vi "multi_line_to_single_line.vi"(0 "input string":string, 11 "error in (no error)":errorcluster) -> (4 "result string":string, 15 "error out":errorcluster)   [LabVIEW 2023]
doc: "Used to convert a multine string to single line string."
uses:
  <vilib>/Utility/error.llb/Trim Whitespace One-Sided.vi
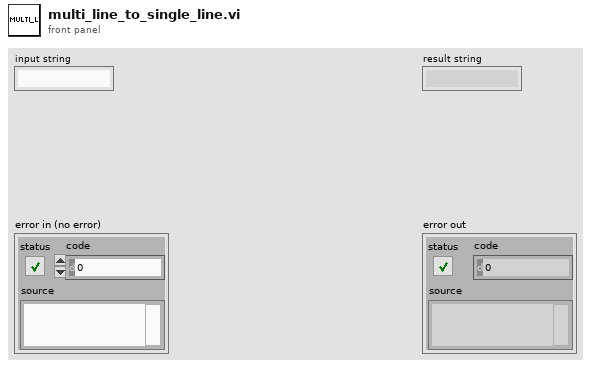
[diagram p1: front panel]
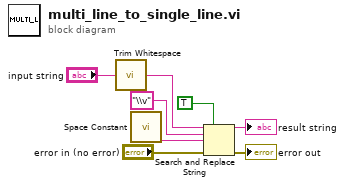
[diagram p0: block diagram]
diagram:
  n1 = call <vilib>:"Trim Whitespace.vi"("string"="input string") -> ("trimmed string"=w2:string)  [unwired: 1 in]
  n2 = call <vilib>:"Space Constant.vi"() -> ("String"=w8:string)
  n3 = Search and Replace String(replace all?=TRUE ("replace all? (F)"), input string=w2, search string="\\v", replace string=w8, error in="error in (no error)") -> (result string=→"result string":string, error out=→"error out":errorcluster)  [unwired: 3 in, 2 out]
